vi "Send REGISTER.vi"(8 "REGISTER request data":T1, 9 "Message Loop Shift Register Data":T2, 10 "error in (no error)":errorcluster, 11 "WAMP Client in":refnum<class "WAMP Client.lvclass">) -> (1 "Message Loop Shift Register Data":T2, 2 "error out":errorcluster, 3 "WAMP Client out":refnum<class "WAMP Client.lvclass">)   [LabVIEW 2020, in "wamplv.lvlib" / "WAMP Client.lvclass"]
uses:
  WAMP Client.lvclass
  TypeDef/Message Loop Shift Reg Data.ctl
  TypeDef/REGISTER Request Data.ctl
  TypeDef/Success or error.ctl
  API/TypeDefs/Combined error.ctl
  API/TypeDefs/WAMP error.ctl
  TypeDef/Publish Requests Map.ctl
  TypeDef/PUBLISH Request Data.ctl
  TypeDef/PUBLISH result.ctl
  TypeDef/Endpoint Data.ctl
  TypeDef/CALL Request Map.ctl
  TypeDef/CALL Request Data.ctl
  API/TypeDefs/RESULT payload.ctl
  TypeDef/SUBSCRIBE Requests Map.ctl
  TypeDef/SUBSCRIBE Request Data.ctl
  TypeDef/Subscribe Result.ctl
  TypeDef/EVENT payload.ctl
  TypeDef/Subscriptions Map.ctl
  TypeDef/Subscription Details.ctl
  TypeDef/Unsubscribe Requests Map.ctl
  TypeDef/UNSUBSCRIBE Request Data.ctl
  TypeDef/UNSUBSCRIBE Result.ctl
  TypeDef/Unregister requests map.ctl
  TypeDef/Unregister request.ctl
  WAMP Client.lvclass/WAMP Client.ctl
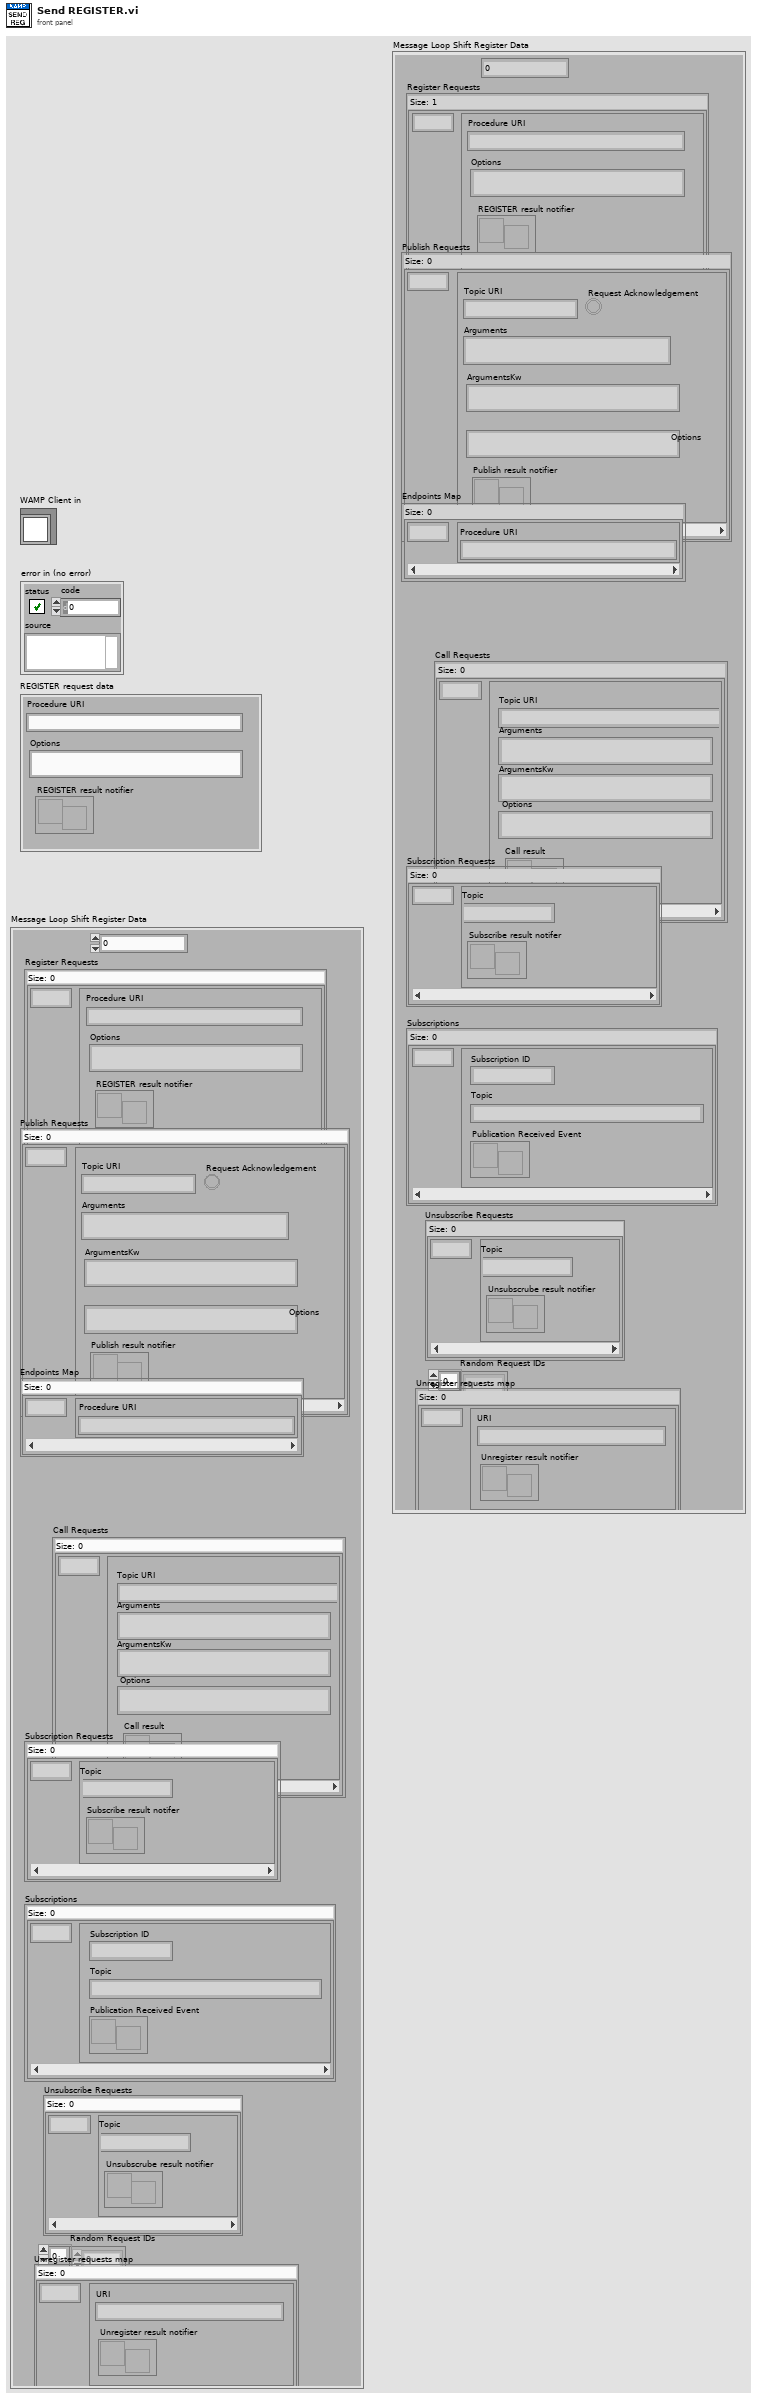
[diagram p1: front panel]
types:
  T1 = typedef "wamplv.lvlib/WAMP Client.lvclass/REGISTER Request Data.ctl" = cluster{"Procedure URI":string, "Options":string, "REGISTER result notifier":refnum<notifier>}
  T2 = typedef "wamplv.lvlib/WAMP Client.lvclass/Message Loop Shift Reg Data.ctl" = cluster{"Last Request ID":u64, "Register Requests":map{u64, T1}, "Publish Requests":T3, "Endpoints Map":map{u64, T5}, "Call Requests":T6, "Subscription Requests":T8, "Subscriptions":T10, "Unsubscribe Requests":T12, "Random Request IDs":u64[], "Unregister requests map":T14}
  T3 = typedef "wamplv.lvlib/WAMP Client.lvclass/Publish Requests Map.ctl" = map{u64, T4}
  T4 = typedef "wamplv.lvlib/WAMP Client.lvclass/PUBLISH Request Data.ctl" = cluster{"Topic URI":string, "Arguments":string, "ArgumentsKw":string, "Request Acknowledgement":bool, "Options":string, "Publish result notifier":refnum<notifier>}
  T5 = typedef "wamplv.lvlib/WAMP Client.lvclass/Endpoint Data.ctl" = cluster{"Procedure URI":string}
  T6 = typedef "wamplv.lvlib/WAMP Client.lvclass/CALL Request Map.ctl" = map{u64, T7}
  T7 = typedef "wamplv.lvlib/WAMP Client.lvclass/CALL Request Data.ctl" = cluster{"Topic URI":string, "Arguments":string, "ArgumentsKw":string, "Options":string, "Call result":refnum<notifier>}
  T8 = typedef "wamplv.lvlib/WAMP Client.lvclass/SUBSCRIBE Requests Map.ctl" = map{u64, T9}
  T9 = typedef "wamplv.lvlib/WAMP Client.lvclass/SUBSCRIBE Request Data.ctl" = cluster{"Topic":string, "Subscribe result notifer":refnum<notifier>}
  T10 = typedef "wamplv.lvlib/WAMP Client.lvclass/Subscriptions Map.ctl" = map{u64, T11}
  T11 = typedef "wamplv.lvlib/WAMP Client.lvclass/Subscription Details.ctl" = cluster{"Subscription ID":u64, "Topic":string, "Publication Received Event":refnum<user-event>}
  T12 = typedef "wamplv.lvlib/WAMP Client.lvclass/Unsubscribe Requests Map.ctl" = map{u64, T13}
  T13 = typedef "wamplv.lvlib/WAMP Client.lvclass/UNSUBSCRIBE Request Data.ctl" = cluster{"Topic":string, "Unsubscrube result notifier":refnum<notifier>}
  T14 = typedef "wamplv.lvlib/WAMP Client.lvclass/Unregister requests map.ctl" = map{u64, T15}
  T15 = typedef "wamplv.lvlib/WAMP Client.lvclass/Unregister request.ctl" = cluster{"URI":string, "Unregister result notifier":refnum<notifier>}
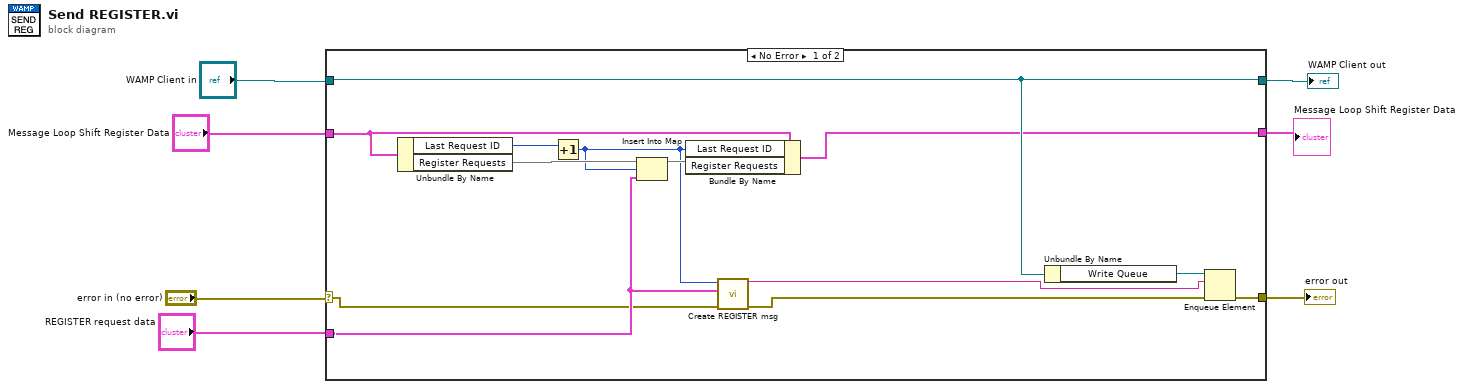
[diagram p0: block diagram]
diagram:
  n1 = case shown="No Error" "error in (no error)" {
    selector: "error in (no error)" -> [w10 w23]
    tunnel: [w17 w23] -> w6
    tunnel: [w18 w22] -> w4
    tunnel: "WAMP Client in" -> [w18 w22]
    tunnel: "REGISTER request data" -> [w14 _]
    tunnel: "Message Loop Shift Register Data" -> [w13 w21]
    tunnel: [w11 w21] -> w1
    frame No Error {
      n2 = Unbundle By Name(w13) -> ("Last Request ID"=w9:u64, "Register Requests"=w15:map{u64, T1})
      n3 = Increment(x=w9) -> (x+1=w8:u64)
      n4 = Insert Into Map(map in=w15, key=w8, value=w14) -> (map out=w12:map{u64, T1})  [unwired: 2 out]
      n5 = Bundle By Name(cluster=w13, "Last Request ID"=w8, "Register Requests"=w12) -> (w11:T2)
      n6 = call "Create REGISTER msg.vi"("error in (no error)"=w10, "REGISTER request data"=w14, "Request  ID"=w8) -> ("error out"=w20:errorcluster, "String"=w19:string)  [unwired: 7 in]
      n7 = Unbundle By Name(w18) -> ("Write Queue"=w16:refnum<queue>)
      n8 = Enqueue Element(queue=w16, element=w19, error in (no error)=w20) -> (error out=w17:errorcluster)  [unwired: 1 in, 2 out]
    }
    frame Error {
    }
  }
  "error out" <- w6
  "WAMP Client out" <- w4
  "Message Loop Shift Register Data" <- w1
